vi "Load Step UI Class.vi"(8 "error in (no error)":errorcluster, 11 "Step Folder Path":path) -> (0 "error out":errorcluster, 2 "Step Name":string, 3 "Step UI out":refnum<class "Step UI.lvclass">)   [LabVIEW 2015, in "Configuration Tool.lvlib"]
uses:
  Configuration Tool.lvlib
  Prototype/classes/Step/UI/Step UI.lvclass
  <vilib>/Utility/error.llb/Error Cluster From Error Code.vi
  <vilib>/ErrorRing/Error Ring.xnode
  <vilib>/NI/Configuration Framework/class discovery singleton/class discovery singleton.lvlib
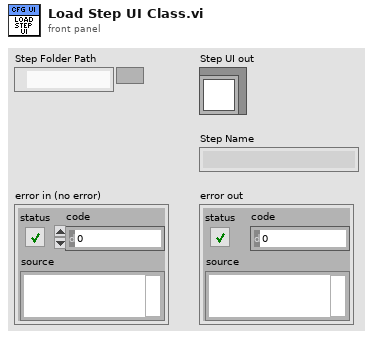
[diagram p1: front panel]
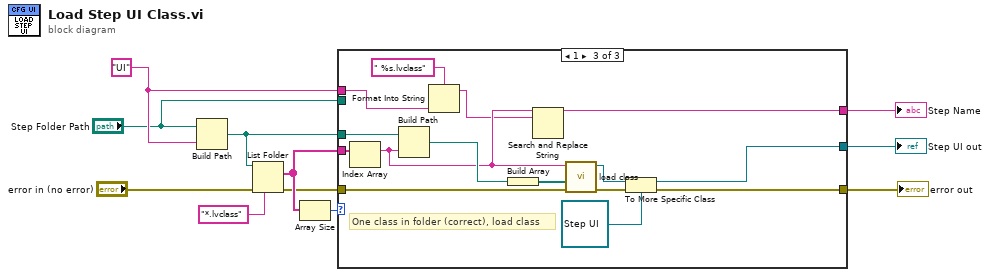
[diagram p0: block diagram]
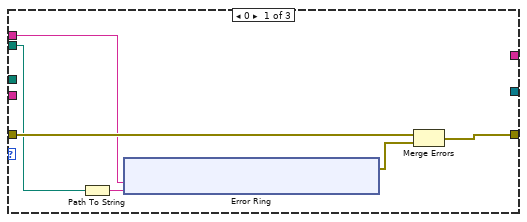
[diagram p2: hidden frame]
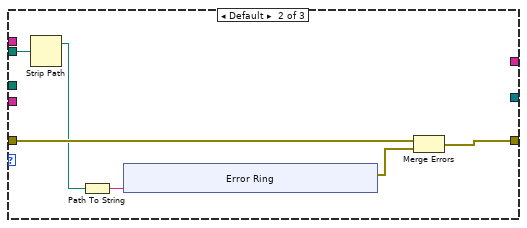
[diagram p3: hidden frame]
diagram:
  w11 = "UI" ("name or relative path")
  n1 = Build Path(base path="Step Folder Path", name or relative path=w11) -> (appended path=w4:path)
  n2 = List Folder(path=w4, pattern="*.lvclass", error in="error in (no error)") -> (filenames=w6:string[], error out=w2:errorcluster)  [unwired: 1 in, 2 out]
  n3 = Array Size(array=w6) -> (size(s)=w7:i32)
  n4 = case shown="1" w7 {
    tunnel: w2 -> [w17 w31 w50]
    tunnel: w4 -> [_ _ w49]
    tunnel: w6 -> [_ _ w48]
    tunnel: [w16 w30 w44] -> w5
    tunnel: "Step Folder Path" -> [w15 w29 _]
    tunnel: [_ _ w43] -> w9
    tunnel: [_ _ w42] -> w10
    tunnel: w11 -> [w12 _ w39]
    frame 0 {
      n5 = Path To String(path=w15) -> (string=w13:string)
      n6 = xnode "Error Ring"("parameter 0"=w12, "parameter 1"=w13) -> ("error out"=w14:errorcluster)
      n7 = Merge Errors(w17, w14) -> (w16:errorcluster)
    }
    frame Default {
      n8 = Strip Path(path=w29) -> (stripped path=w28:path)  [unwired: 1 out]
      n9 = Path To String(path=w28) -> (string=w27:string)
      n10 = xnode "Error Ring"("parameter 0"=w27) -> ("error out"=w26:errorcluster)
      n11 = Merge Errors(w31, w26) -> (w30:errorcluster)
    }
    frame 1 {
      # "One class in folder (correct), load class"
      n12 = Index Array(array=w48) -> (element=w45:string)  [unwired: 1 in]
      n13 = Build Path(base path=w49, name or relative path=w45) -> (appended path=w47:path)
      n14 = Format Into String(format string=" %s.lvclass" ("search string"), w39) -> (resulting string=w40:string)  [unwired: 2 in, 1 out]
      n15 = Build Array(w47) -> (w46:path[])
      n16 = Search and Replace String(input string=w45, search string=w40) -> (result string=w43:string)  [unwired: 6 in, 3 out]
      n17 = call <vilib>:"load class.vi"("error in"=w50, "available class paths"=w46, "Class Name"=w45) -> ("error out"=w51:errorcluster, "Object Out"=w53:refnum<class>)  [unwired: 7 in]
      n18 = To More Specific Class(target class=refnum<class "Step UI.lvclass"> refnum ("Step UI.lvclass"), reference=w53, error in=w51) -> (specific class reference=w42:refnum<class "Step UI.lvclass">, error out=w44:errorcluster)
    }
  }
  "Step UI out" <- w10
  "Step Name" <- w9
  "error out" <- w5
